vi "BRig_RT_comm_webdav_upload_all.vi"(0 "input_I_connected_webdav":bool, 1 "input_fileName_prefix":string, 5 "input_hSession":T1, 7 "input_error":errorcluster) -> (6 "output_hSession":T1, 8 "error out":errorcluster, 12 "output_nFilenames":i32, 13 "output_arrFilenames":string[](array[string]), 14 "output_uploaded":bool[](array[boolean]), 15 "output_strCmd":string)   [LabVIEW 2014]
uses:
  <vilib>/WebDAVClient/Advanced/SessionHandle.ctl
  <vilib>/WebDAVClient/NI_WebDAV.lvlib
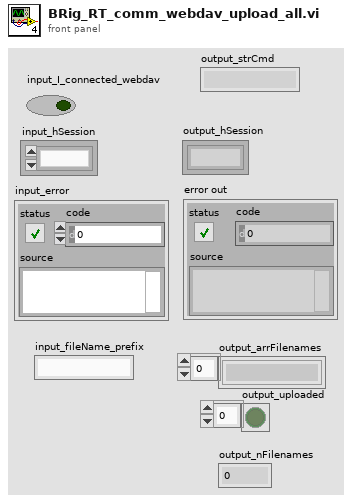
[diagram p1: front panel]
types:
  T1 = typedef "NI_WebDAV.lvlib/SessionHandle.ctl" = refnum<k1>
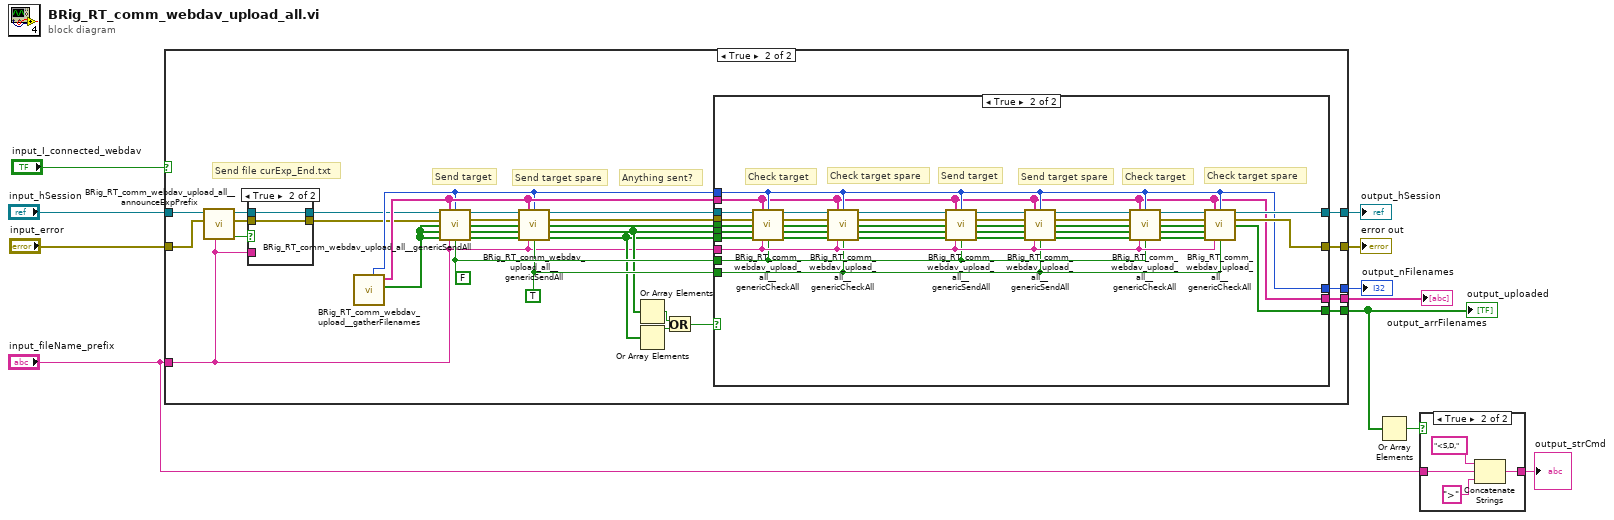
[diagram p0: block diagram]
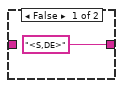
[diagram p2: hidden frame]
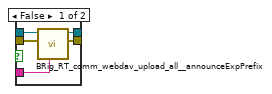
[diagram p4: hidden frame]
diagram:
  n1 = case shown="True" "input_I_connected_webdav" {
    tunnel: "input_hSession" -> [w13 w21]
    tunnel: [w13 w26] -> w9
    tunnel: "input_error" -> [w12 w20]
    tunnel: [w12 w25] -> w7
    tunnel: "input_fileName_prefix" -> [_ w16]
    tunnel: [_ w24] -> w5
    tunnel: [_ w23] -> w6
    tunnel: [_ w22] -> w4
    frame False {
    }
    frame True {
      w34 = TRUE ("input_Target(F)_or_Spare(T)")
      w35 = FALSE ("input_Target(F)_or_Spare(T)")
      # "Send file curExp_End.txt"
      # "Anything sent?"
      # "Send target spare"
      # "Send target"
      n2 = call "BRig_RT_comm_webdav_upload_all__announceExpPrefix.vi"("input_fileName_prefix"=w16, "input_errro"=w20, "intput_hSession"=w21) -> ("output_checkData"=w17:bool, "output_error"=w18:errorcluster, "output_hSession"=w19:T1)  [unwired: 6 in]
      n3 = case shown="True" w17 {
        tunnel: w19 -> [w49 w51]
        tunnel: w18 -> [w48 w50]
        tunnel: w16 -> [w47 _]
        tunnel: [w46 w51] -> w15
        tunnel: [w45 w50] -> w14
        frame False {
          n4 = call "BRig_RT_comm_webdav_upload_all__announceExpPrefix.vi"("input_fileName_prefix"=w47, "input_errro"=w48, "intput_hSession"=w49) -> ("output_error"=w45:errorcluster, "output_hSession"=w46:T1)  [unwired: 6 in, 1 out]
        }
        frame True {
        }
      }
      n5 = call "BRig_RT_comm_webdav_upload__gatherFilenames.vi"() -> ("output_arrBlank"=w44:bool[], "output_arrFilenames"=w33:string[], "output_n"=w32:i32)  [unwired: 9 in]
      n6 = call "BRig_RT_comm_webdav_upload_all__genericSendAll.vi"("input_hSession"=w15, "input_arrFilenames"=w33, "input_n"=w32, "input_error"=w14, "input_arrUploaded"=w44, "input_arrSentTarget"=w44, "input_arrSentTargetSpare"=w44, "input_fileName_prefix"=w16, "input_Target(F)_or_Spare(T)"=w35) -> ("output_hSession"=w43:T1, "output_error"=w42:errorcluster, "output_arrUploaded"=w41:bool[], "output_arrSentTarget"=w40:bool[], "output_arrSentTargetSpare"=w39:bool[])  [unwired: 2 in]
      n7 = call "BRig_RT_comm_webdav_upload_all__genericSendAll.vi"("input_hSession"=w43, "input_arrFilenames"=w33, "input_n"=w32, "input_error"=w42, "input_arrUploaded"=w41, "input_arrSentTarget"=w40, "input_arrSentTargetSpare"=w39, "input_fileName_prefix"=w16, "input_Target(F)_or_Spare(T)"=w34) -> ("output_hSession"=w38:T1, "output_error"=w37:errorcluster, "output_arrUploaded"=w36:bool[], "output_arrSentTarget"=w31:bool[], "output_arrSentTargetSpare"=w30:bool[])  [unwired: 2 in]
      n8 = Or Array Elements(Boolean array=w31) -> (logical OR=w28:bool)
      n9 = Or Array Elements(Boolean array=w30) -> (logical OR=w29:bool)
      n10 = Or(x=w28, y=w29) -> (x .or. y?=w27:bool)
      n11 = case shown="True" w27 {
        tunnel: w38 -> [w56 w94]
        tunnel: w37 -> [w55 w93]
        tunnel: w36 -> [w52 w92]
        tunnel: w35 -> [_ w63]
        tunnel: w16 -> [_ w64]
        tunnel: w34 -> [_ w62]
        tunnel: w33 -> [w53 w57]
        tunnel: w32 -> [w54 w58]
        tunnel: w31 -> [_ w86]
        tunnel: w30 -> [_ w85]
        tunnel: [w56 w61] -> w26
        tunnel: [w55 w60] -> w25
        tunnel: [w54 w58] -> w24
        tunnel: [w53 w57] -> w23
        tunnel: [w52 w59] -> w22
        frame False {
        }
        frame True {
          # "Check target spare"
          # "Check target"
          # "Send target spare"
          # "Send target"
          # "Check target spare"
          # "Check target"
          n12 = call "BRig_RT_comm_webdav_upload_all__genericCheckAll.vi"("input_hSession"=w94, "input_arrFilenames"=w57, "input_n"=w58, "input_error"=w93, "input_arrUploaded"=w92, "input_arrSentTarget"=w86, "input_arrSentTargetSpare"=w85, "input_fileName_prefix"=w64, "input_Target(F)_or_Spare(T)"=w63) -> ("output_hSession"=w91:T1, "output_error"=w90:errorcluster, "output_arrUploaded"=w89:bool[], "output_arrSentTarget"=w88:bool[], "output_arrSentTargetSpare"=w87:bool[])  [unwired: 2 in]
          n13 = call "BRig_RT_comm_webdav_upload_all__genericCheckAll.vi"("input_hSession"=w91, "input_arrFilenames"=w57, "input_n"=w58, "input_error"=w90, "input_arrUploaded"=w89, "input_arrSentTarget"=w88, "input_arrSentTargetSpare"=w87, "input_fileName_prefix"=w64, "input_Target(F)_or_Spare(T)"=w62) -> ("output_hSession"=w84:T1, "output_error"=w83:errorcluster, "output_arrUploaded"=w82:bool[], "output_arrSentTarget"=w81:bool[], "output_arrSentTargetSpare"=w80:bool[])  [unwired: 2 in]
          n14 = call "BRig_RT_comm_webdav_upload_all__genericSendAll.vi"("input_hSession"=w84, "input_arrFilenames"=w57, "input_n"=w58, "input_error"=w83, "input_arrUploaded"=w82, "input_arrSentTarget"=w81, "input_arrSentTargetSpare"=w80, "input_fileName_prefix"=w64, "input_Target(F)_or_Spare(T)"=w63) -> ("output_hSession"=w79:T1, "output_error"=w78:errorcluster, "output_arrUploaded"=w77:bool[], "output_arrSentTarget"=w76:bool[], "output_arrSentTargetSpare"=w75:bool[])  [unwired: 2 in]
          n15 = call "BRig_RT_comm_webdav_upload_all__genericSendAll.vi"("input_hSession"=w79, "input_arrFilenames"=w57, "input_n"=w58, "input_error"=w78, "input_arrUploaded"=w77, "input_arrSentTarget"=w76, "input_arrSentTargetSpare"=w75, "input_fileName_prefix"=w64, "input_Target(F)_or_Spare(T)"=w62) -> ("output_hSession"=w74:T1, "output_error"=w72:errorcluster, "output_arrUploaded"=w71:bool[], "output_arrSentTarget"=w70:bool[], "output_arrSentTargetSpare"=w69:bool[])  [unwired: 2 in]
          n16 = call "BRig_RT_comm_webdav_upload_all__genericCheckAll.vi"("input_hSession"=w74, "input_arrFilenames"=w57, "input_n"=w58, "input_error"=w72, "input_arrUploaded"=w71, "input_arrSentTarget"=w70, "input_arrSentTargetSpare"=w69, "input_fileName_prefix"=w64, "input_Target(F)_or_Spare(T)"=w63) -> ("output_hSession"=w73:T1, "output_error"=w68:errorcluster, "output_arrUploaded"=w67:bool[], "output_arrSentTarget"=w66:bool[], "output_arrSentTargetSpare"=w65:bool[])  [unwired: 2 in]
          n17 = call "BRig_RT_comm_webdav_upload_all__genericCheckAll.vi"("input_hSession"=w73, "input_arrFilenames"=w57, "input_n"=w58, "input_error"=w68, "input_arrUploaded"=w67, "input_arrSentTarget"=w66, "input_arrSentTargetSpare"=w65, "input_fileName_prefix"=w64, "input_Target(F)_or_Spare(T)"=w62) -> ("output_hSession"=w61:T1, "output_error"=w60:errorcluster, "output_arrUploaded"=w59:bool[])  [unwired: 2 in, 2 out]
        }
      }
    }
  }
  "error out" <- w7
  "output_hSession" <- w9
  "output_arrFilenames" <- w6
  "output_nFilenames" <- w5
  "output_uploaded" <- w4
  n18 = Or Array Elements(Boolean array=w4) -> (logical OR=w3:bool)
  n19 = case shown="True" w3 {
    tunnel: "input_fileName_prefix" -> [_ w97]
    tunnel: ["<S,DE>" ("string") w96] -> w1
    frame False {
    }
    frame True {
      n20 = Concatenate Strings("<S,D," ("string"), w97, ">" ("string")) -> (w96:string)
    }
  }
  "output_strCmd" <- w1
